vi "CPP_Aeroprobe_TimeSeries-Array.vi"() -> (5 "Plug in titles":string[](array[string]), 7 "Plug in values":string[](array[string]))   [LabVIEW 2013]
uses:
  Globals/Meas_global.vi
panel:
  out "AvgReduction (ms)":dbl
  out "reduction ms":u32
  in  "Calibration Folder Path":path=path "M:/Preferences/Rig_Setups/All_Rigs/Calibrations/5HoleProbe"
  in  "Correction File Path":path=path "M:/Preferences/Rig_Setups/All_Rigs/TubingCompensation/5HPTubingCorrection12066.xls"
  in  "Apply Phase Correction?":bool=TRUE
  out "DataArray":dbl[](array[numeric])
  out "Zeroes":dbl[](array[numeric])
  # "!! 5-hole 1-5 must be connected to Channels 1-5 !!"
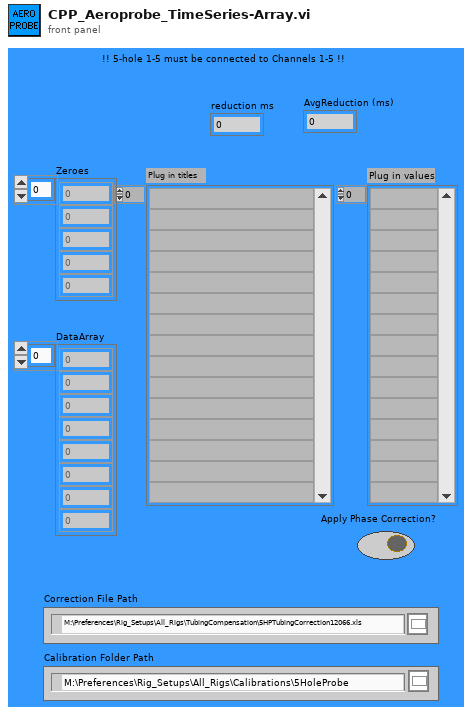
[diagram p1: front panel]
types:
  T1 = typedef "Analysis_info_cluster.ctl" = cluster{"Colour":u32, "Inst type":T2, "Inst name":string, "Symbol":string, "Code name":string, "Extra Info":string, "Inst Array":T3, "Extra Titles":string[], "Extra Values":string[], "U":dbl, "u^2":dbl, "u^3":dbl, "u^4":dbl, "Skew_u":dbl, "Kurt_u":dbl, "Sd Error in Mean":dbl, "% u'/U":dbl, "X":dbl, "Y":dbl, "Z":dbl, "Timescale integral to 25%":dbl, "Sd Error in Variance":dbl, "Calib File":path, "Calib Constants":dbl[], "Output Position":bool, "Full Stats":bool, "Av Sampling Rate":dbl, "Av No of Samples":dbl, "Total Meas Time (s)":dbl, "ADAM Ch Name":string}
  T2 = typedef "Inst_type.ctl" = enum16{"Propeller anemometer", "Raw voltage", "Pressure Transducer", "Pitot-static tube", "Preston tube", "Hot wire", "Cross wire 1", "Cross wire 2", "Generic Linear", "Generic Polynomial", "Generic BackPoly", "Fast FID", "Thermocouple", "Cold wire", "Pulsed Wire", "LDA Vel", "LDA Tran time", "LDA Arr time"}
  T3 = typedef "Instrument_Array.ctl" = enum16{"PWA", "LDA", "Analogue"}
  T4 = cluster{"Analysis Info cluster[0]":T1, "Analysis Info cluster[1]":T1, "Analysis Info cluster[2]":T1, "Analysis Info cluster[3]":T1, "Analysis Info cluster[4]":T1, "Analysis Info cluster[5]":T1, "Analysis Info cluster[6]":T1}
  T5 = typedef "Time_Trace_Cluster.ctl" = cluster{"Weighting":dbl[], "Time (s)":dbl[], "Voltage":dbl[], "Eng Values":dbl[]}
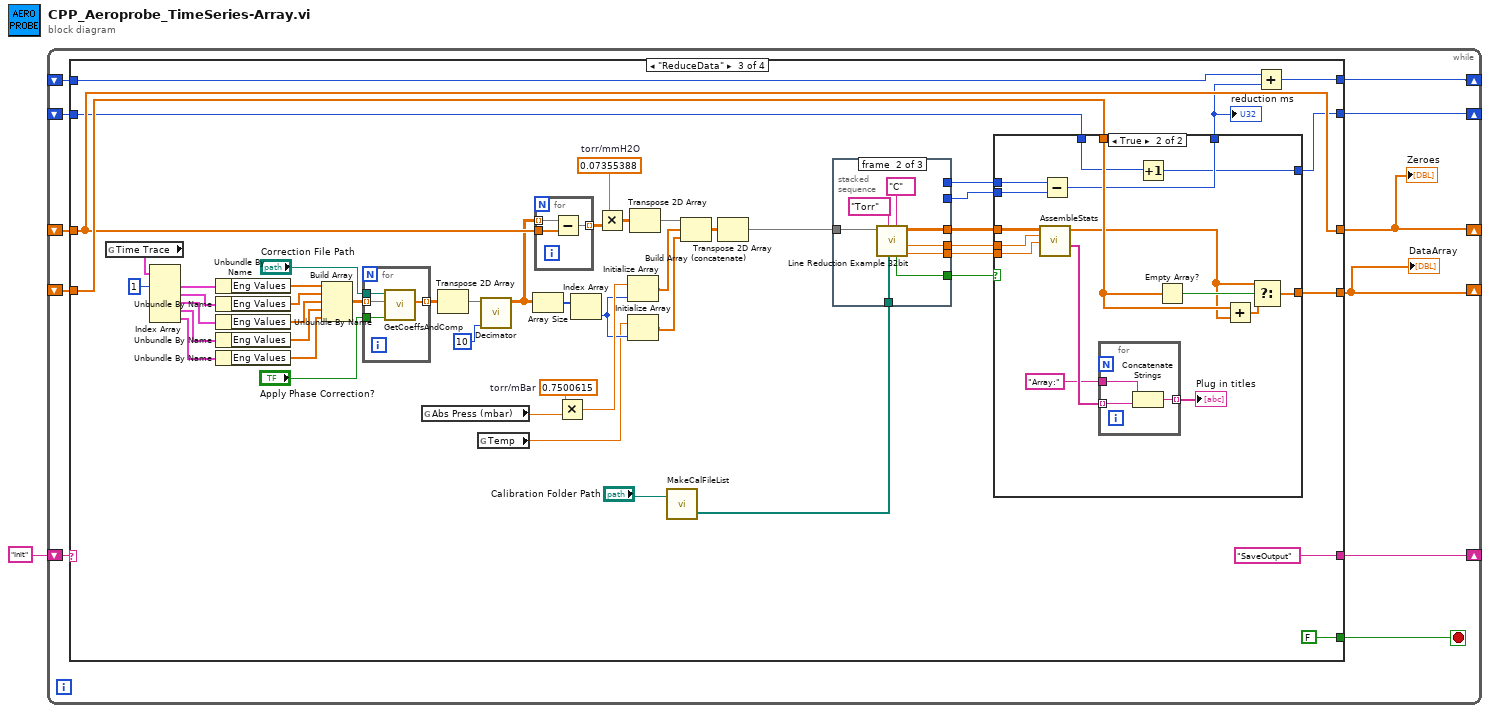
[diagram p0: block diagram]
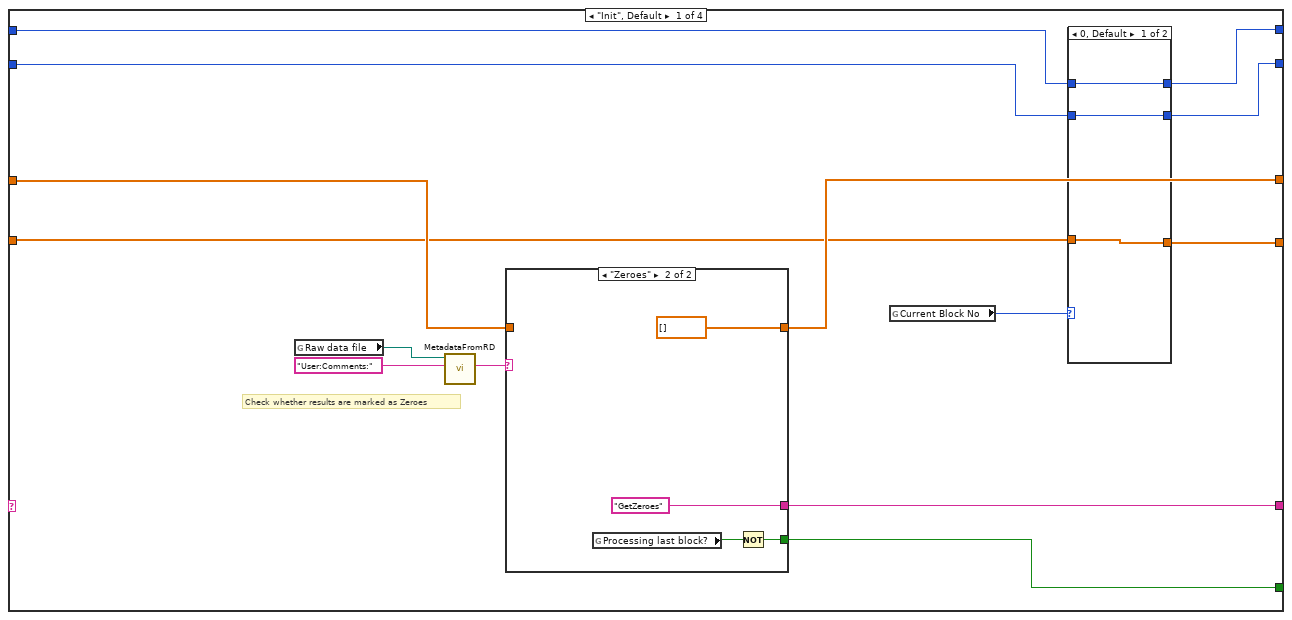
[diagram p2: hidden frame]
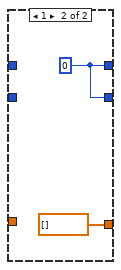
[diagram p3: hidden frame]
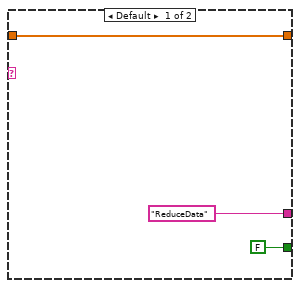
[diagram p4: hidden frame]
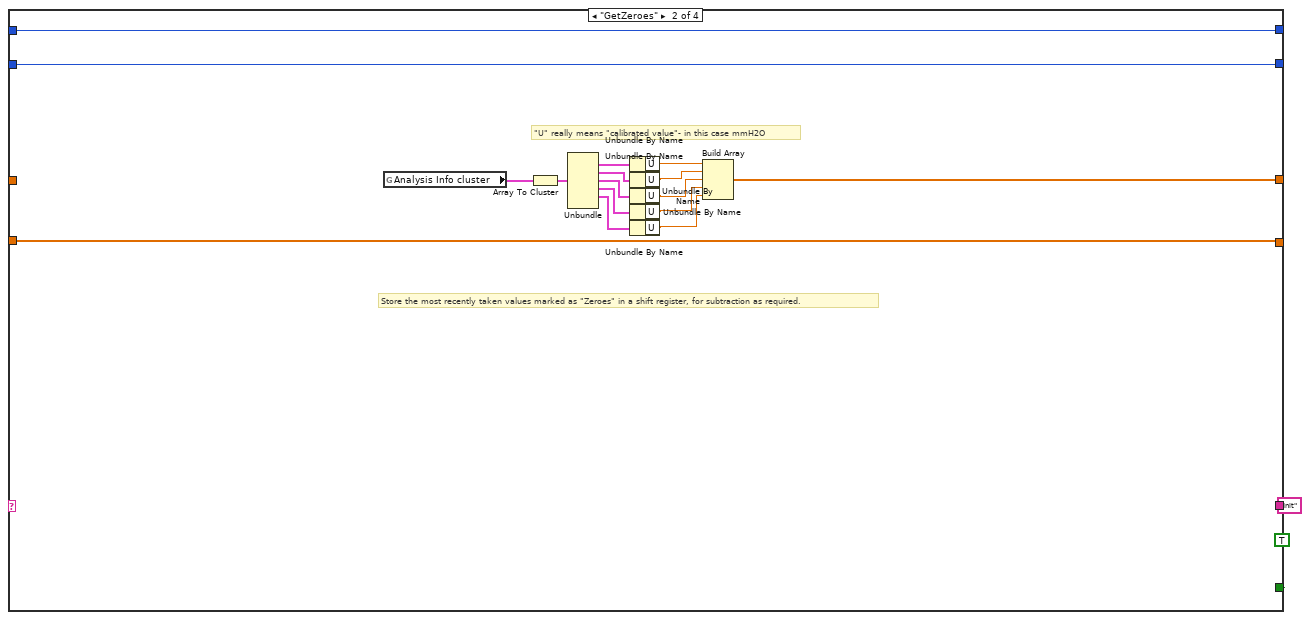
[diagram p5: hidden frame]
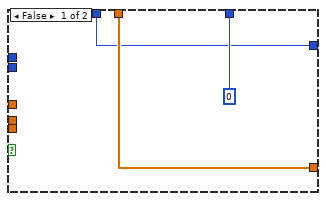
[diagram p6: hidden frame]
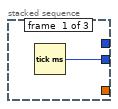
[diagram p7: hidden frame]
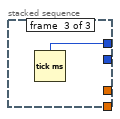
[diagram p8: hidden frame]
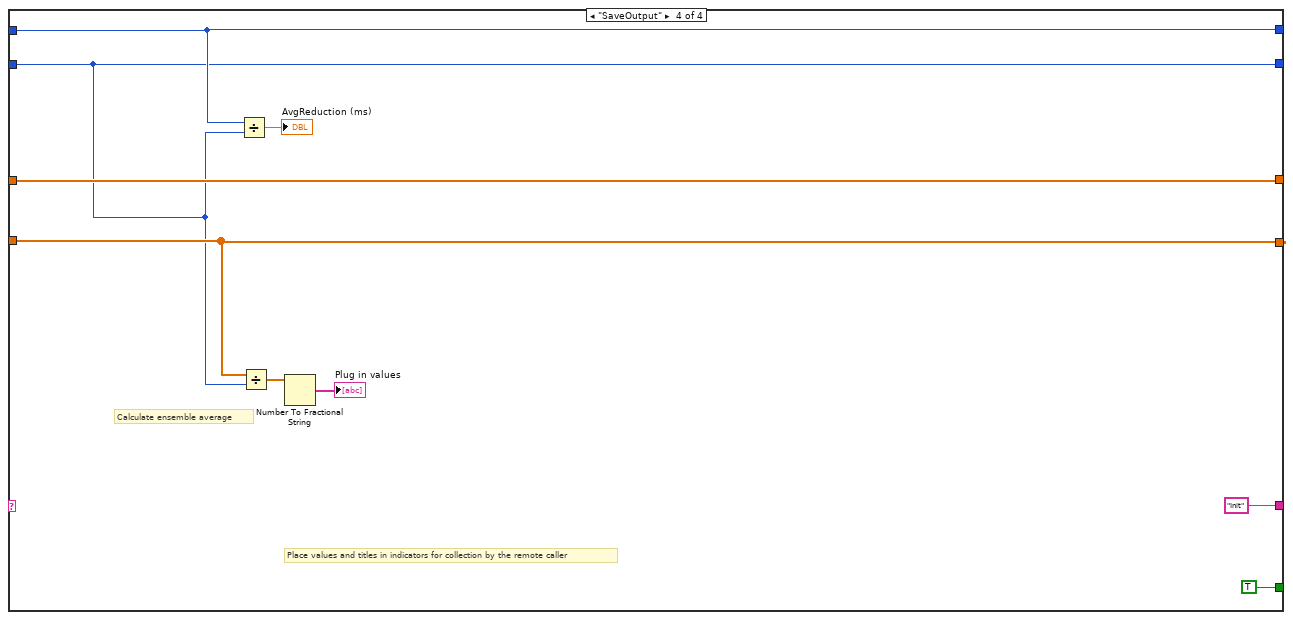
[diagram p9: hidden frame]
diagram:
  n1 = while {
    shift-right: [w11] -> _
    shift-left: "Init" -> [w12]
    shift-right: [w10] -> _
    shift-left: _ -> [w9]
    shift-right: [w8] -> _
    shift-left: _ -> [w7]
    shift-right: [w5] -> _
    shift-left: _ -> [w4]
    shift-right: [w2] -> _
    shift-left: _ -> [w3]
    stop <- w6 stop-if-true
    n2 = case shown="\"ReduceData\"" w12 {
      tunnel: [w26 "Init" "SaveOutput" "Init"] -> w11
      tunnel: [w20 w43 w82 w155] -> w10
      tunnel: w9 -> [w21 _ w82 w155]
      tunnel: [w18 w41 w92 w151] -> w8
      tunnel: w7 -> [w17 w41 w93 w151]
      tunnel: [w22 TRUE FALSE TRUE] -> w6
      tunnel: [w16 w40 w67 w149] -> w5
      tunnel: w4 -> [w14 w40 w65 w149]
      tunnel: w3 -> [w13 w39 w58 w147]
      tunnel: [w15 w39 w57 w147] -> w2
      frame "Init", Default {
        # "Check whether results are marked as Zeroes"
        n3 = global read "Meas_global.vi" "Raw data file"() -> (w25:path)
        n4 = call "MetadataFromRD.vi"("ChannelName"="User:Comments:", "Raw data file"=w25) -> ("ValueString"=w23:string)  [unwired: 8 in, 1 out]
        n5 = case shown="\"Zeroes\"" w23 {
          tunnel: ["ReduceData" "GetZeroes"] -> w26
          tunnel: [FALSE w37] -> w22
          tunnel: w21 -> [w32 _]
          tunnel: [w32 dbl[] [] ("t")] -> w20
          frame Default {
          }
          frame "Zeroes" {
            n6 = global read "Meas_global.vi" "Processing last block?"() -> (w36:bool)
            n7 = Not(x=w36) -> (.not. x?=w37:bool)
          }
        }
        n8 = global read "Meas_global.vi" "Current Block No"() -> (w19:i32)
        n9 = case shown="0, Default" w19 {
          tunnel: [w29 dbl[] [] ("t")] -> w18
          tunnel: w17 -> [w29 _]
          tunnel: [w28 w30] -> w16
          tunnel: [w27 w30] -> w15
          tunnel: w14 -> [w28 _]
          tunnel: w13 -> [w27 _]
          frame 0, Default {
          }
          frame 1 {
            w30 = u32 0
          }
        }
      }
      frame "GetZeroes" {
        # "Store the most recently taken values marked as \"Zeroes\" in a shift register, for subtraction as required."
        # "\"U\" really means \"calibrated value\"- in this case mmH2O"
        n10 = global read "Meas_global.vi" "Analysis Info cluster"() -> (w45:T1[])
        n11 = Array To Cluster(array=w45) -> (cluster=w51:T4)
        n12 = Unbundle(w51) -> ("Analysis Info cluster[1]"=w52:T1, "Analysis Info cluster[2]"=w53:T1, "Analysis Info cluster[3]"=w54:T1, "Analysis Info cluster[4]"=w55:T1, "Analysis Info cluster[5]"=w56:T1)  [unwired: 2 out]
        n13 = Unbundle By Name(w52) -> ("U"=w50:dbl)
        n14 = Unbundle By Name(w53) -> ("U"=w49:dbl)
        n15 = Unbundle By Name(w54) -> ("U"=w48:dbl)
        n16 = Unbundle By Name(w55) -> ("U"=w47:dbl)
        n17 = Unbundle By Name(w56) -> ("U"=w46:dbl)
        n18 = Build Array(w50, w49, w48, w47, w46) -> (w43:dbl[])
      }
      frame "ReduceData" {
        w85 = 0.07355388  # torr/mmH2O
        w86 = 0.7500615  # torr/mBar
        n19 = global read "Meas_global.vi" "Time Trace"() -> (w97:T5[])
        n20 = Index Array(array=w97, index #1=1 ("index")) -> (element #1=w96:T5, element #2=w105:T5, element #3=w104:T5, element #4=w103:T5, element #5=w102:T5)  [unwired: 4 in]
        n21 = Unbundle By Name(w96) -> ("Eng Values"=w95:dbl[])
        n22 = Unbundle By Name(w105) -> ("Eng Values"=w101:dbl[])
        n23 = Unbundle By Name(w104) -> ("Eng Values"=w100:dbl[])
        n24 = Unbundle By Name(w103) -> ("Eng Values"=w99:dbl[])
        n25 = Unbundle By Name(w102) -> ("Eng Values"=w98:dbl[])
        n26 = Build Array(w95, w101, w100, w99, w98) -> (w91:dbl[][])
        n27 = for {
          tunnel: w91 -> [w146] mode=indexing
          tunnel: [w145] -> w88 mode=indexing
          tunnel: "Apply Phase Correction?" -> [w144]
          tunnel: "Correction File Path" -> [w143]
          n28 = call "GetCoeffsAndComp.vi"("Apply Phase Correction?"=w144, "mutedData"=w146, "TubingCorrectionFile (pre-set!)"=w143) -> ("boostedData"=w145:dbl[])  [unwired: 8 in]
        }
        n29 = global read "Meas_global.vi" "Abs Press (mbar)"() -> (w87:dbl)
        n30 = Transpose 2D Array(2D array=w88) -> (transposed array=w69:dbl[][])
        n31 = global read "Meas_global.vi" "Temp"() -> (w71:dbl)
        n32 = call "Decimator.vi"("Divider"=10, "Array In"=w69) -> ("Array Out"=w68:dbl[][])  [unwired: 9 in]
        n33 = Array Size(array=w68) -> (size(s)=w81:i32[])
        n34 = for {
          tunnel: [w142] -> w84 mode=indexing
          tunnel: w68 -> [w141] mode=indexing
          tunnel: w82 -> [w140]
          n35 = Subtract(x=w141, y=w140) -> (x-y=w142:dbl[])
        }
        n36 = Multiply(x=w86, y=w87) -> (x*y=w80:dbl)
        n37 = Index Array(array=w81) -> (element=w79:i32)  [unwired: 1 in]
        n38 = Multiply(x=w85, y=w84) -> (x*y=w78:dbl[][])
        n39 = Initialize Array(w80, w79) -> (w76:dbl[])
        n40 = Initialize Array(w71, w79) -> (w75:dbl[])
        n41 = Transpose 2D Array(2D array=w78) -> (transposed array=w73:dbl[][])
        n42 = call "MakeCalFileList.vi"("Calibration Folder Path"="Calibration Folder Path") -> ("Calibration File(s)"=w74:path[])  [unwired: 1 in, 1 out]
        n43 = Build Array (concatenate)(w73, w76, w75) -> (w77:dbl[][])
        n44 = Transpose 2D Array(2D array=w77) -> (transposed array=w72:dbl[][])
        n45 = stacked-sequence {
          tunnel: w72 -> [_ w137 _]
          tunnel: w74 -> [_ w138 _]
          tunnel: [w130 _ _] -> w64
          tunnel: [_ _ w139] -> w63
          tunnel: [_ w134 _] -> w62
          tunnel: [_ w133 _] -> w61
          tunnel: [_ w132 _] -> w60
          tunnel: [_ w131 _] -> w59
          frame #0 {
            n46 = Tick Count (ms)() -> (millisecond timer value=w130:u32)
          }
          frame #1 {
            n47 = call "Line Reduction Example 32bit.vi"("Temperature Units"="C", "Calibration File(s)"=w138, "Pressure Units"="Torr", "Data to Reduce"=w137) -> ("MyConeExceededFraction"=w132:dbl, "GoodFraction"=w133:dbl, "VmagUVWCone"=w134:dbl[][], "GoodBlock"=w131:bool)  [unwired: 4 in]
          }
          frame #2 {
            n48 = Tick Count (ms)() -> (millisecond timer value=w139:u32)
          }
        }
        n49 = case shown="True" w59 {
          tunnel: w93 -> [w110 w126]
          tunnel: [w110 w123] -> w92
          tunnel: [u32 0 w122] -> w66
          tunnel: w64 -> [_ w121]
          tunnel: w63 -> [_ w120]
          tunnel: w62 -> [_ w119]
          tunnel: w61 -> [_ w118]
          tunnel: w60 -> [_ w117]
          tunnel: w58 -> [w108 w115]
          tunnel: [w108 w114] -> w57
          frame False {
          }
          frame True {
            n50 = call "AssembleStats.vi"("ExcessiveConeFraction"=w117, "ValidFraction"=w118, "VmagUVWCone"=w119) -> ("Plug in titles"=w113:string[], "StatsArray"=w116:dbl[])  [unwired: 7 in]
            n51 = Subtract(x=w120, y=w121) -> (x-y=w122:u32)
            n52 = for {
              tunnel: w113 -> [w129] mode=indexing
              tunnel: "Array:" -> [w128]
              tunnel: [w127] -> w111 mode=indexing
              n53 = Concatenate Strings(w128, w129) -> (w127:string)
            }
            "Plug in titles" <- w111
            n54 = Increment(x=w115) -> (x+1=w114:u32)
            n55 = Empty Array?(array=w126) -> (empty?=w125:bool)
            n56 = Add(x=w126, y=w116) -> (x+y=w124:dbl[])
            n57 = Select(t=w116, s=w125, f=w124) -> (s? t:f=w123:dbl[])
          }
        }
        "reduction ms" <- w66
        n58 = Add(x=w65, y=w66) -> (x+y=w67:u32)
      }
      frame "SaveOutput" {
        # "Place values and titles in indicators for collection by the remote caller"
        # "Calculate ensemble average"
        n59 = Divide(x=w149, y=w147) -> (x/y=→"AvgReduction (ms)":dbl)
        n60 = Divide(x=w151, y=w147) -> (x/y=w150:dbl[])
        n61 = Number To Fractional String(number=w150) -> (F-format string=→"Plug in values":string[])  [unwired: 3 in]
      }
    }
    "Zeroes" <- w10
    "DataArray" <- w8
  }
